vi "Read single frame from binary file.vi"(8 "error in (no error)":errorcluster, 10 "Frame position in Cam binary file":i64, 11 "Binary video ref":refnum<file>) -> (0 "error out":errorcluster, 1 "Rel time (ms)":u32, 2 "Image":T1(plugin-control), 3 "Binary video ref":refnum<file>)   [LabVIEW 2020]
uses:
  Typedefs/Binary Cam data type definition.ctl
  <vilib>/vision/Image Controls.llb/IMAQ Image.ctl
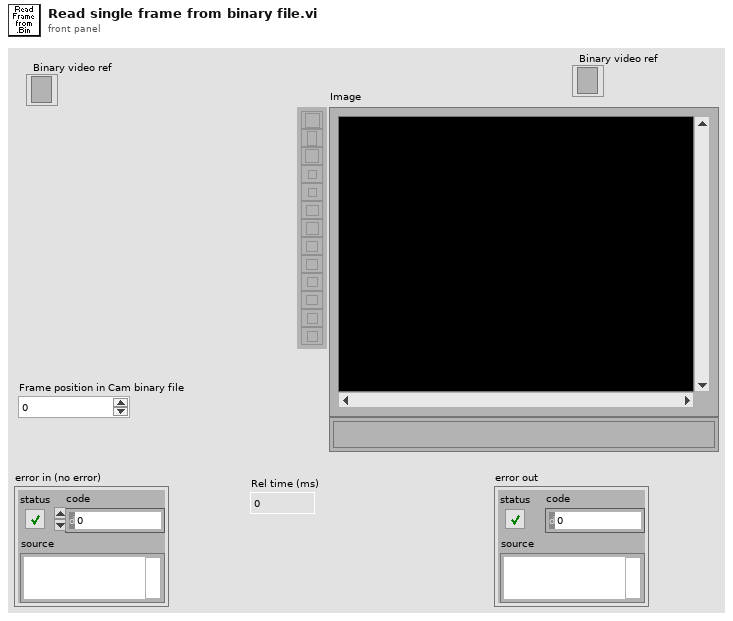
[diagram p1: front panel]
types:
  T1 = typedef "IMAQ Image.ctl" = refnum<image>
  T2 = typedef "Binary Cam data type definition.ctl" = cluster{"Image":T1, "Rel time":u32}
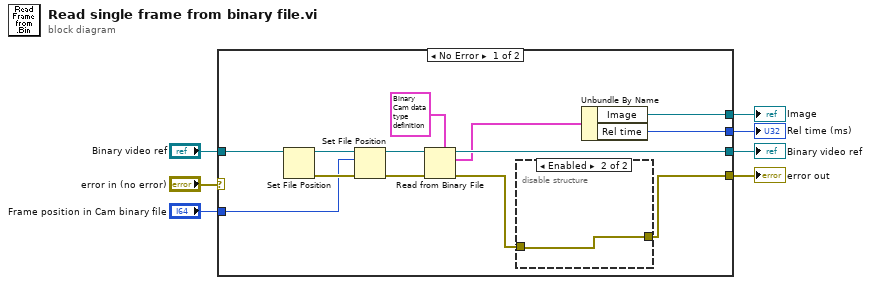
[diagram p0: block diagram]
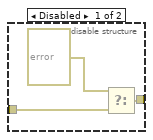
[diagram p2: hidden frame]
diagram:
  n1 = case shown="No Error" "error in (no error)" {
    selector: "error in (no error)" -> [_ w26]
    tunnel: [w10 w26] -> w6
    tunnel: "Binary video ref" -> [w17 w25]
    tunnel: "Frame position in Cam binary file" -> [w14 _]
    tunnel: [w12 _] -> w2
    tunnel: [w11 _] -> w3
    tunnel: [w9 w25] -> w1
    frame No Error {
      n2 = Set File Position(refnum=w17) -> (refnum out=w19:refnum<file>, error out=w18:errorcluster)  [unwired: 3 in]
      n3 = Set File Position(offset (in bytes) (0)=w14, refnum=w19, error in=w18) -> (refnum out=w16:refnum<file>, error out=w15:errorcluster)  [unwired: 1 in]
      n4 = Read from Binary File(5:T2 {"Image"=refnum, "Rel time"=0} ("output cluster"), 8:w15, 11:w16) -> (0:w13:errorcluster, 2:w8:T2, 3:w9:refnum<file>)  [unwired: 3 in, 1 out]
      n5 = disable-structure shown="Enabled" {
        disable-tunnel: w13 -> [w23 w24]
        disable-tunnel: [w21 w24] -> w10
        frame Disabled {
          n6 = Select(t=errorcluster {"status"=TRUE, "code"=5001, "source"="Data array read from binary video file is empty"} ("error out"), f=w23) -> (s? t:f=w21:errorcluster)  [unwired: 1 in]
        }
        frame Enabled {
        }
      }
      n7 = Unbundle By Name(w8) -> ("Image"=w12:T1, "Rel time"=w11:u32)
    }
    frame Error {
    }
  }
  "error out" <- w6
  "Rel time (ms)" <- w3
  "Image" <- w2
  "Binary video ref" <- w1
